vi "NHR_Initialize.vi"(2 "NHR error in":errorcluster caption="error in (no error)", 3 "NHR VISA":refnum<visa-resource-name>) -> (0 "NHR error out":errorcluster, 1 "NHR VISA out":refnum<visa-resource-name>)   [LabVIEW 2020]
uses:
  <instrlib>/NH Research Regenerative Test Series/NH Research Regenerative Test Series.lvlib
panel:
  in  "Logical Instrument Number":u32=1
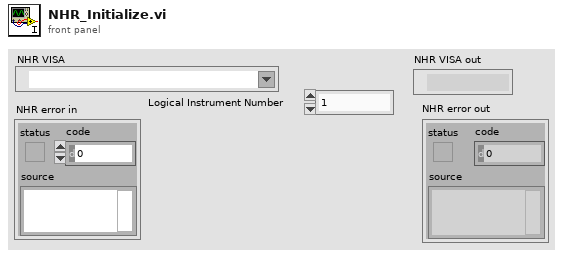
[diagram p1: front panel]
types:
  T1 = cluster{"Min Voltage (V)":dbl, "Min Voltage Time (s)":dbl, "Max Voltage (V)":dbl, "Max Voltage Time (s)":dbl, "Max Sink Current (A)":dbl, "Max Sink Current Time (s)":dbl, "Max Source Current (A)":dbl, "Max Source Current Time (s)":dbl, "Max Sink Power (W)":dbl, "Max Sink Power Time (s)":dbl, "Max Source Power (W)":dbl, "Max Source Power Time (s)":dbl}
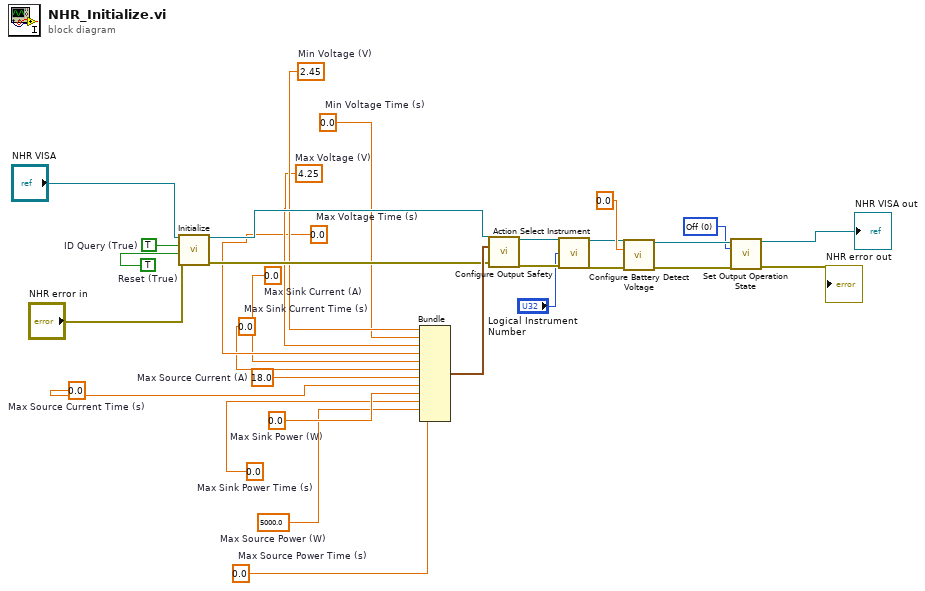
[diagram p0: block diagram]
diagram:
  w4 = 0 items=["Off", "Standby", "Charge", "Discharge", "Battery"] ("Mode (0: Off)")
  w23 = TRUE  # ID Query (True)
  w22 = TRUE  # Reset (True)
  w11 = 5000.0  # Max Source Power (W)
  w12 = 0.0  # Max Sink Power Time (s)
  w13 = 0.0  # Max Sink Power (W)
  w14 = 0.0  # Max Source Current Time (s)
  w15 = 18.0  # Max Source Current (A)
  w17 = 0.0  # Max Sink Current (A)
  w16 = 0.0  # Max Sink Current Time (s)
  w18 = 0.0  # Max Voltage Time (s)
  w19 = 4.25  # Max Voltage (V)
  w21 = 2.45  # Min Voltage (V)
  w10 = 0.0  # Max Source Power Time (s)
  w20 = 0.0  # Min Voltage Time (s)
  n1 = call <instrlib>:"Initialize.vi"("VISA resource name"="NHR VISA", "ID Query (True)"=w23, "Reset (True)"=w22, "error in (no error)"="NHR error in") -> ("VISA resource name out"=w25:refnum<visa-resource-name>, "error out"=w26:errorcluster)  [unwired: 10 in]
  n2 = Bundle("Min Voltage (V)"=w21, "Min Voltage Time (s)"=w20, "Max Voltage (V)"=w19, "Max Voltage Time (s)"=w18, "Max Sink Current (A)"=w17, "Max Sink Current Time (s)"=w16, "Max Source Current (A)"=w15, "Max Source Current Time (s)"=w14, "Max Sink Power (W)"=w13, "Max Sink Power Time (s)"=w12, "Max Source Power (W)"=w11, "Max Source Power Time (s)"=w10) -> (w27:T1)  [unwired: 1 in]
  n3 = call <instrlib>:"Configure Output Safety.vi"("VISA resource name"=w25, "Output Safety"=w27, "error in (no error)"=w26) -> ("VISA resource name out"=w29:refnum<visa-resource-name>, "error out"=w30:errorcluster)  [unwired: 11 in]
  n4 = call <instrlib>:"Action Select Instrument.vi"("VISA resource name"=w29, "Logical Instrument Number"="Logical Instrument Number", "error in (no error)"=w30) -> ("VISA resource name out"=w8:refnum<visa-resource-name>, "error out"=w7:errorcluster)  [unwired: 11 in]
  n5 = call <instrlib>:"Configure Battery Detect Voltage.vi"("VISA resource name"=w8, "Battery Detect Voltage (0V)"=0.0, "error in (no error)"=w7) -> ("VISA resource name out"=w6:refnum<visa-resource-name>, "error out"=w5:errorcluster)  [unwired: 11 in]
  n6 = call <vilib>:"Set Output Operation State.vi"("VISA resource name"=w6, "Mode (0: Off)"=w4, "error in (no error)"=w5) -> ("VISA resource name out"=→"NHR VISA out":refnum<visa-resource-name>, "error out"=→"NHR error out":errorcluster)  [unwired: 11 in]
